vi "Template - Scope Acquire Waveform Continuously.vi"() -> ()   [LabVIEW 2020]
doc: "This example shows how to use autosetup and acquire a waveform continuously on a single channel.\n\n<B>Note:</B> In this example, each record is acquired independently and not as a continuous stream of data."
uses:
  <instrlib>/_Template - Scope/Public/Data/Read Waveform (Single).vi
  <instrlib>/_Template - Scope/Template - Scope.lvlib
panel:
  in  "Maximum Time (10000 ms)":u32=10000
  in  "Serial Configuration":T1={"Baud Rate"=9600, "Parity"=0, "Data Bits"=7, "Stop Bits"=10, "Flow Control"=0} {"Flow Control" items=["None", "XON/XOFF", "RTS/CTS", "XON/XOFF & RTS/CTS", "DTR/DSR", "XON/XOFF & DTR/DSR"]; "Stop Bits" items=["1.0"=10, "1.5"=15, "2.0"=20]; "Data Bits" items=["7"=7, "8"=8]; "Parity" items=["None", "Odd", "Even", "Mark", "Space"]; "Baud Rate" items=["300"=300, "600"=600, "1200"=1200, "2400"=2400, "4800"=4800, "9600"=9600, "19200"=19200]}
  in  "stop":bool
  in  "Probe Attenuation (10.0)":dbl=10.0
  out "Waveform Data":waveform(dbl)(graph)
  in  "Channel (1: Channel 1)":u16(ring)=1 items=["Channel 1"=1, "Channel 2"=2]
  in  "VISA resource name":refnum<visa-resource-name>
  # "(c) 2014 <Enter Company Name Here>.  ALL RIGHTS RESERVED."
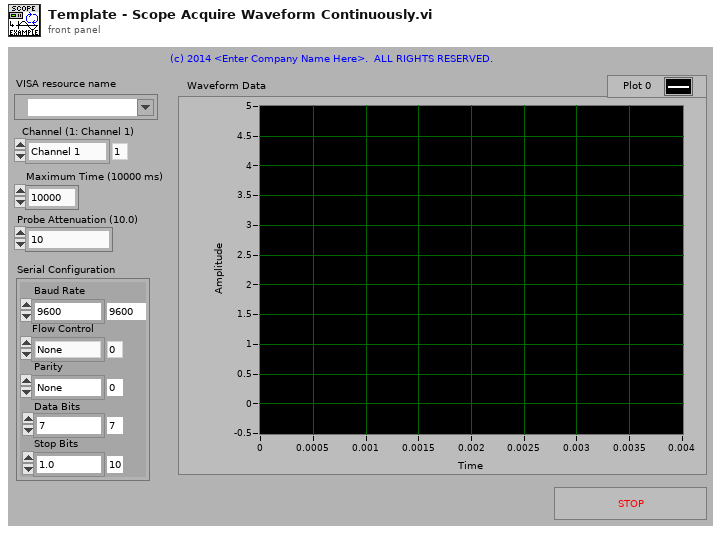
[diagram p1: front panel]
types:
  T1 = cluster{"Baud Rate":u32, "Parity":u16, "Data Bits":u16, "Stop Bits":u16, "Flow Control":u16}
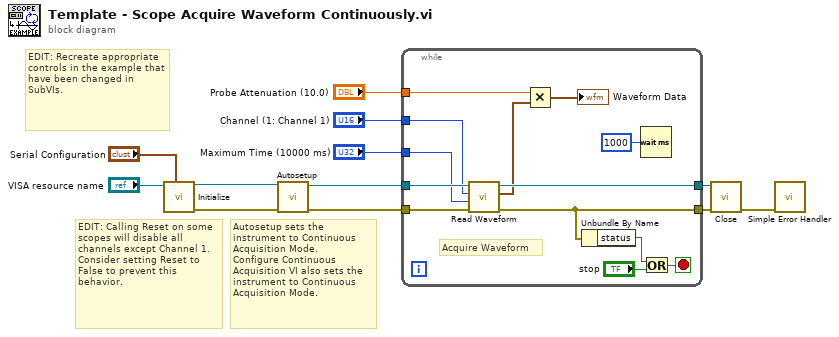
[diagram p0: block diagram]
diagram:
  # "EDIT: Calling Reset on some scopes will disable all channels except Channel 1. Consider setting Reset to False to prevent this behavior."
  # "EDIT: Recreate appropriate controls in the example that have been changed in SubVIs."
  # "Autosetup sets the instrument to Continuous Acquisition Mode.\nConfigure Continuous Acquisition VI also sets the instrument to Continuous Acquisition Mode."
  n1 = call <instrlib>:"Initialize.vi"("Serial Configuration"="Serial Configuration", "VISA resource name"="VISA resource name") -> ("error out"=w7:errorcluster, "VISA resource name out"=w6:refnum<visa-resource-name>)  [unwired: 8 in]
  n2 = call <instrlib>:"Autosetup.vi"("error in (no error)"=w7, "VISA resource name"=w6) -> ("error out"=w3:errorcluster, "VISA resource name out"=w4:refnum<visa-resource-name>)  [unwired: 8 in]
  n3 = while {
    tunnel: w4 -> [w19]
    tunnel: w3 -> [w14]
    tunnel: [w18] -> w11
    tunnel: [w13] -> w10
    tunnel: "Channel (1: Channel 1)" -> [w15]
    tunnel: "Probe Attenuation (10.0)" -> [w25]
    tunnel: "Maximum Time (10000 ms)" -> [w16]
    stop <- w22 stop-if-true
    # "Acquire Waveform"
    n4 = call-poly <instrlib>:"Read Waveform.vi"("error in (no error)"=w14, "Maximum Time (10000 ms)"=w16, "Channel (1: Channel 1)"=w15, "VISA resource name"=w19) -> ("error out"=w13:errorcluster, "Waveform Data"=w17:waveform(dbl), "VISA resource name out"=w18:refnum<visa-resource-name>)  [unwired: 5 in]
    n5 = Multiply(x=w25, y=w17) -> (x*y=→"Waveform Data":waveform(dbl))
    n6 = Unbundle By Name(w13) -> ("status"=w21:bool)
    n7 = Wait (ms)(milliseconds to wait=u32 1000 ("millisecond multiple")) -> ()  [unwired: 1 out]
    n8 = Or(x=w21, y="stop") -> (x .or. y?=w22:bool)
  }
  n9 = call <instrlib>:"Close.vi"("error in (no error)"=w10, "VISA resource name"=w11) -> ("error out"=w12:errorcluster)  [unwired: 9 in]
  n10 = call <vilib>:"Simple Error Handler.vi"("error in (no error)"=w12) -> ()  [unwired: 4 in, 5 out]
